vi "Write DbConnection.vi"(8 "error in (no error)":errorcluster, 10 "Dapper.lvlib:DbConnection.lvclass":refnum<class "DbConnection.lvclass">, 11 "SqlMapper in":refnum<class "SqlMapper.lvclass">) -> (0 "error out":errorcluster, 3 "SqlMapper out":refnum<class "SqlMapper.lvclass">)   [LabVIEW 2020, in "ORM.lvlib" / "SqlMapper.lvclass"]
uses:
  SqlMapper.lvclass
  DbConnection/DbConnection.lvclass
  SqlMapper.lvclass/SqlMapper.ctl
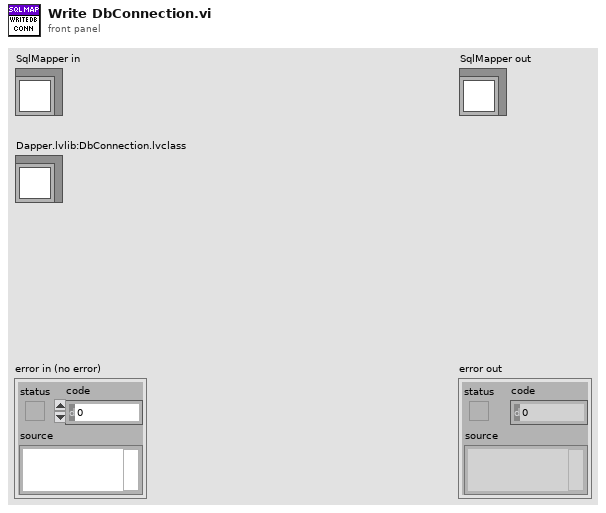
[diagram p1: front panel]
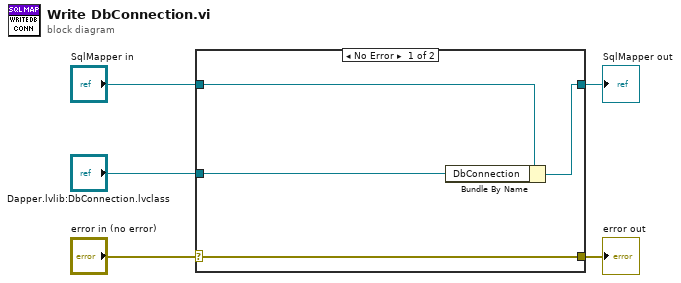
[diagram p0: block diagram]
diagram:
  n1 = case shown="No Error" "error in (no error)" {
    selector: "error in (no error)" -> [w9 w10]
    tunnel: [w9 w10] -> w4
    tunnel: [w7 w11] -> w2
    tunnel: "SqlMapper in" -> [w8 w11]
    tunnel: "Dapper.lvlib:DbConnection.lvclass" -> [w6 _]
    frame No Error {
      n2 = Bundle By Name(cluster=w8, "DbConnection"=w6) -> (w7:refnum<class "SqlMapper.lvclass">)
    }
    frame Error {
    }
  }
  "error out" <- w4
  "SqlMapper out" <- w2
